vi "InitDataRaw.vi"(7 "Get/Set":T2, 11 "MomentValues in":T1) -> (3 "MomentValues Out":T1)   [LabVIEW 2019]
uses:
  Communication/TypeDef/#TypeDef_SetGet.ctl
  TypeDef/#TypeDef_MomentValues.ctl
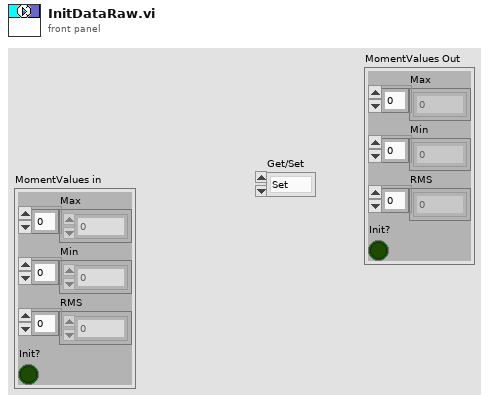
[diagram p1: front panel]
types:
  T1 = typedef "#TypeDef_MomentValues.ctl" = cluster{"Max":dbl[], "Min":dbl[], "RMS":dbl[], "Init?":bool}
  T2 = typedef "#TypeDef_SetGet.ctl" = enum16{"Set", "Get"}
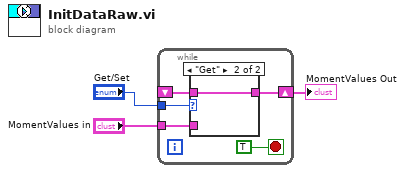
[diagram p0: block diagram]
diagram:
  n1 = while {
    tunnel: "Get/Set" -> [w7]
    shift-right: [w4] -> w1
    shift-left: _ -> [w6]
    tunnel: "MomentValues in" -> [w5]
    stop <- TRUE stop-if-true
    n2 = case shown="\"Get\"" w7 {
      tunnel: w6 -> [_ w10]
      tunnel: w5 -> [w9 _]
      tunnel: [w9 w10] -> w4
      frame "Set", Default {
      }
      frame "Get" {
      }
    }
  }
  "MomentValues Out" <- w1
